vi "tkrsa6100 Spectrum Msmt Results.vi"(0 "VISA Resource Name":refnum<visa-resource-name>, 1 "Byte Count\n(100000)":i32=100000 min=10000 max=1000000 step=1000, 5 "Run Acquisition and/or \nGet Result (RUN ACQUISITION & GET RESULT)":T1(ring), 7 "Spectrum Trace(1)":enum16{"1", "2", "3", "MATH", "SGRAM"}(ring), 9 "Timeout (S)\n(30)":i32=30 min=1 max=1000 step=1, 11 "error in (no error)":errorcluster {"code" format="%#.0f"}, 12 "Convert Resp\nString(NO)":enum16{"NO", "YES"}(ring)) -> (4 "dup VISA Resource Name":refnum<visa-resource-name>, 6 "Measurement\nResponse String":string, 8 "# Data Points":i32, 10 "Converted Sgl Float\nResponse String":string, 15 "error out":errorcluster {"code" format="%#.0f"})   [LabVIEW 2020, in "Library Instrument & Equipement.lvlib" / "Library Spectrum Analyser.lvlib"]
doc: "Prerequisites for use:\n \nThis VI is valid in the Spectrum Analysis measurement view in the General Signal Viewing measurement group.\n\nThis VI controls the following functions.\nRetrieves all Spectrum Analyzer traces.\n\nerror in (no error) is checked by tkrsa6100 Write/Read wError Query.vi for any pending errors.\n\nIf error in status is ERROR:\n\nerror in (no error) and VISA Resource Name are passed straight through to error out and dup VISA Resource Name of the Write/Read Drivers and returned to the calling function. No commands are processed.\n\nIf error in status is NO ERROR:\n\nPass the following functions to enumerated control Run Acquisition and/or Get Result (RUN ACQUISITION & GET RESULT).\n\nRUN ACQUISITION & GET RESULT\nRuns an acquisition and retrieves the trace data. Additionally this function puts the instrument into single acquisition mode.\n\nGET LAST ACQUISITION RESULT\nRetrieves the last acquired trace data.\n\nAlso pass the following items.\n\nSpectrumTrace (1)\nSelects trace 1, 2, 3, Math Trace, or Spectrogram (SGRAM) trace.\n\nNote: For Spectrogram to be a valid trace, the Spectrogram measurment must be running with the Spectrum measurement.\n\nConvert Resp String (NO)\nPass YES to convert the binary trace data to a comma separated list of single precision floats. This conversion is accomplished by tkrsa6100 Binary String Converter.vi. The precision of the converted floats is set to 12 digits so that values can be displayed in Watts and Volts vertical units.\n\nTimeout (S) (30)\nThis defaults to 30 seconds which should be adequate for most applications. If not pass the desired timeout in seconds.\n\nByte Count (100000)\nThis defaults to 100,000 bytes which should be adequate for most applications. If the entire block is not retrieved increase the count to the desired value.\n\nOne command/query is executed per VI call.\n\nThe format of the returned binary string is:\n\n<#><num digits in num bytes><num bytes><binary block consisting of num bytes of data in 4 byte little-endian format>\n\nInformation returned by the VI is:\n\ndup VISA Resource Name\nError Out\n\nMeasurement Response String. Binary trace data\n\nConverted Sgl Float Response String. Comma separated list of single precision floats converted from the binary data. If Convert Response String is selected as NO this indicator is wired an empty string constant.\n\n# Data Points. Number of actual display points returned. Equal to num bytes/4. If Convert Response String is selected as NO this indicator is wired to a constant 0.\n\nThe appropriate command/query string is passed to tkrsa6100 Write/Read wError Query.vi. VI Input Error Query? is set to YES so query SYST:ERR? is appended to the command string and any current error information is displayed in cluster Error Out. VI Input Response String Format (ASCII) is wired to constant BINARY to handle the binary block.\nOn completion dup VISA Resource Name, Error Out, and Measurement Response String are returned to the calling function."
uses:
  Library Spectrum Analyser.lvlib
panel:
  # "RSA6100 Spectrum Msmt Result Driver"
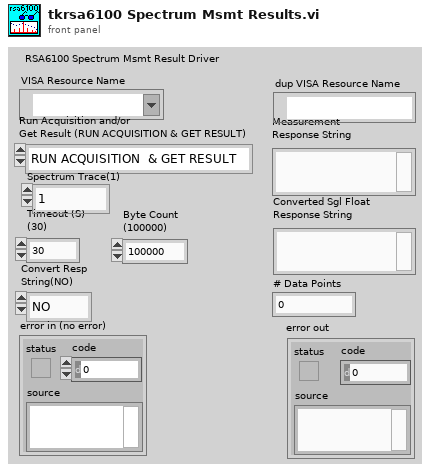
[diagram p1: front panel]
types:
  T1 = enum16{"RUN ACQUISITION  & GET RESULT", "GET LAST ACQUISITION RESULT"}
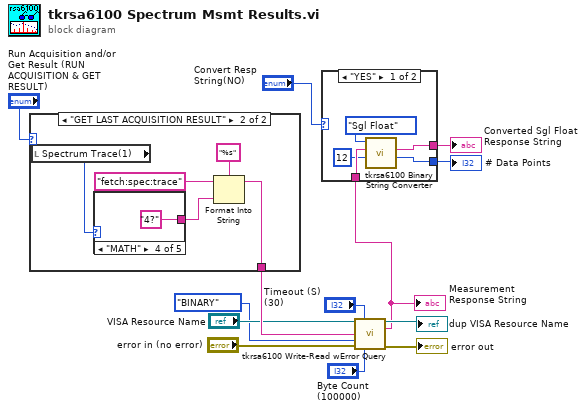
[diagram p0: block diagram]
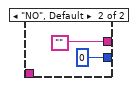
[diagram p2: hidden frame]
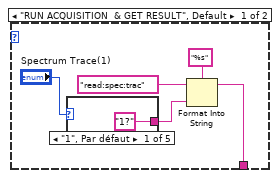
[diagram p3: hidden frame]
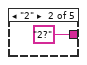
[diagram p4: hidden frame]
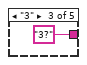
[diagram p5: hidden frame]
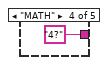
[diagram p6: hidden frame]
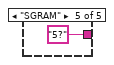
[diagram p7: hidden frame]
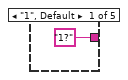
[diagram p8: hidden frame]
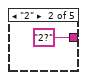
[diagram p9: hidden frame]
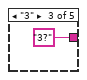
[diagram p10: hidden frame]
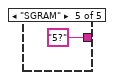
[diagram p11: hidden frame]
diagram:
  n1 = case shown="\"GET LAST ACQUISITION RESULT\"" "Run Acquisition and/or \nGet Result (RUN ACQUISITION & GET RESULT)" {
    tunnel: [w14 w25] -> w9
    frame "RUN ACQUISITION  & GET RESULT", Default {
      n2 = case shown="\"1\", Par défaut" "Spectrum Trace(1)" {
        tunnel: ["1?" ("Command") "2?" ("Command") "3?" ("Command") "4?" ("Command") "5?" ("Command")] -> w15
        frame "1", Default {
        }
        frame "2" {
        }
        frame "3" {
        }
        frame "MATH" {
        }
        frame "SGRAM" {
        }
      }
      n3 = Format Into String(format string="%s", initial string="read:spec:trac" ("Command"), w15) -> (resulting string=w14:string)  [unwired: 1 in, 1 out]
    }
    frame "GET LAST ACQUISITION RESULT" {
      n4 = local read "Spectrum Trace(1)"() -> (w26:enum16{"1", "2", "3", "MATH", "SGRAM"})
      n5 = case shown="\"MATH\"" w26 {
        tunnel: ["1?" ("Command") "2?" ("Command") "3?" ("Command") "4?" ("Command") "5?" ("Command")] -> w27
        frame "1", Default {
        }
        frame "2" {
        }
        frame "3" {
        }
        frame "MATH" {
        }
        frame "SGRAM" {
        }
      }
      n6 = Format Into String(format string="%s", initial string="fetch:spec:trace" ("Command"), w27) -> (resulting string=w25:string)  [unwired: 1 in, 1 out]
    }
  }
  n7 = call "tkrsa6100 Write-Read wError Query.vi"("VISA Resource Name"="VISA Resource Name", "Max Read Byte\nCount (1000)"="Byte Count\n(100000)", "Command (Empty String)"=w9, "Response String \nFormat(ASCII)"=enum16{"ASCII", "BINARY"}."BINARY" ("Response String \nFormat(ASCII)"), "error in (no error)"="error in (no error)", "Timeout(S) (10)"="Timeout (S)\n(30)") -> ("dup VISA Resource Name"=→"dup VISA Resource Name":refnum<visa-resource-name>, "Response"=w8:string, "error out"=→"error out":errorcluster)  [unwired: 1 in, 6 out]
  "Measurement\nResponse String" <- w8
  n8 = case shown="\"YES\"" "Convert Resp\nString(NO)" {
    tunnel: w8 -> [w38 _]
    tunnel: [w37 ""] -> w1
    tunnel: [w36 u32 0 ("# Points")] -> w11
    frame "YES" {
      n9 = call "tkrsa6100 Binary String Converter.vi"("Digits of Precision\n(0)"=u32 12 ("Digits of Precision"), "Binary Msmt Result String\n(Empty String)"=w38, "Data Type\n(Sgl Float)"=enum16{"Sgl Float", "32 Integer"}."Sgl Float" ("Data Type")) -> ("# Points"=w36:i32, "Converted Result String"=w37:string)  [unwired: 7 out]
    }
    frame "NO", Default {
    }
  }
  "Converted Sgl Float\nResponse String" <- w1
  "# Data Points" <- w11
